vi "Terminal-ModbusEthernet-ReadRegistersWithDateTime.vi"(5 "write operation timeout (ms)":i32=5000 caption="写操作超时（毫秒）", 7 "read operation timeout (ms)":i32=5000 caption="读操作超时（毫秒）", 8 "error in":errorcluster, 9 "number of holding registers":u16 caption="保持寄存器数量", 10 "starting address":u16 caption="起始地址", 11 "unit ID":u8 caption="单元ID") -> (0 "error out":errorcluster, 2 "时间标识":timestamp, 3 "register values":u16[](array[numeric]) caption="寄存器值")   [LabVIEW 2014]
uses:
  <vilib>/Modbus/subvis/Modbus API/Modbus API.lvclass/Modbus API.ctl
  <vilib>/Modbus/subvis/Transmission Data Unit (ADU)/Transmission Data Unit/Transmission Data Unit.lvclass/Transmission Data Unit.ctl
  <vilib>/Modbus/master/Data Access/Unit ID/Set Unit ID Property.vi
  <vilib>/Modbus/subvis/Transmission Data Unit (ADU)/Transmission Data Unit/Data Access/Unit ID/Write Unit ID.vi
  <vilib>/Modbus/subvis/Modbus API/Read Transmission Data Unit.vi
  <vilib>/Modbus/subvis/Modbus API/Write Transmission Data Unit.vi
  Configuration-Global.vi
  <vilib>/Modbus/master/Create Master Instance (TCP).vi
  <vilib>/Modbus/subvis/Transmission Data Unit (ADU)/Transmission Data Unit/Transmission Data Unit.lvclass
  <vilib>/Modbus/master/Modbus Master.lvclass
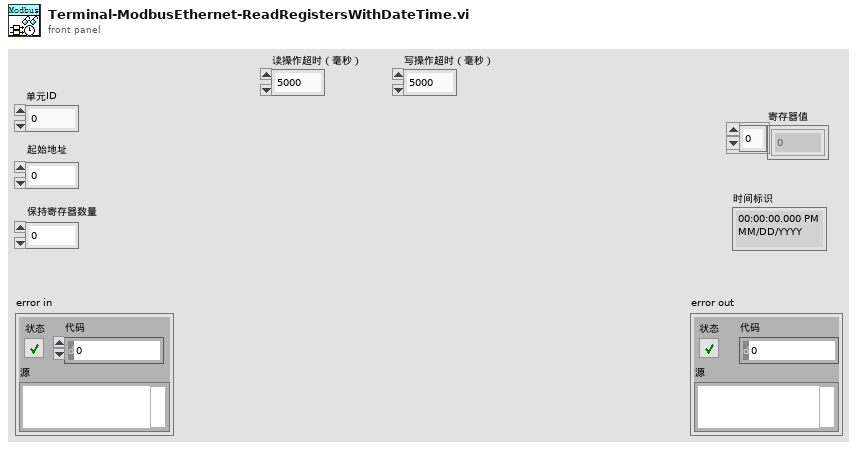
[diagram p1: front panel]
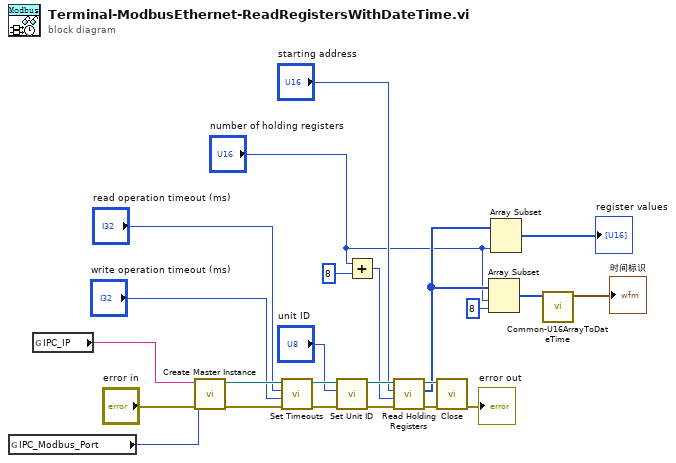
[diagram p0: block diagram]
diagram:
  n1 = global read "Configuration-Global.vi" "IPC_Modbus_Port"() -> (w1:i32)
  n2 = global read "Configuration-Global.vi" "IPC_IP"() -> (w2:string)
  n3 = call-poly <vilib>:"Create Master Instance.vi"("error in (no error)"="error in", "port (502)"=w1, "address"=w2) -> ("error out"=w22:errorcluster, "TCP master instance"=w21:refnum<class "Modbus Master.lvclass">)  [unwired: 7 in]
  n4 = call <vilib>:"Set Timeouts.vi"("error in (no error)"=w22, "write operation timeout (ms)"="write operation timeout (ms)", "read operation timeout (ms)"="read operation timeout (ms)", "Modbus master in"=w21) -> ("error out"=w13:errorcluster, "Modbus master out"=w23:refnum<class "Modbus Master.lvclass">)  [unwired: 6 in]
  n5 = call <vilib>:"Set Unit ID.vi"("error in (no error)"=w13, "unit ID"="unit ID", "Modbus master in"=w23) -> ("error out"=w15:errorcluster, "Modbus master out"=w14:refnum<class "Modbus Master.lvclass">)  [unwired: 7 in]
  n6 = Add(x="number of holding registers", y=u16 8) -> (x+y=w9:u16)
  n7 = call-dynamic "Read Holding Registers.vi"("error in (no error)"=w15, "number of holding registers"=w9, "starting address"="starting address", "Modbus master in"=w14) -> ("error out"=w17:errorcluster, "register values"=w7:u16[], "Modbus master out"=w18:refnum<class "Modbus Master.lvclass">)  [unwired: 5 in]
  n8 = call-dynamic "Close.vi"("error in (no error)"=w17, "Modbus master in"=w18) -> ("error out"=→"error out":errorcluster)  [unwired: 9 in]
  n9 = Array Subset(array=w7, index="number of holding registers", length=8 ("长度")) -> (w4:u16[])
  n10 = Array Subset(array=w7, length="number of holding registers") -> (→"register values":u16[])  [unwired: 1 in]
  n11 = call "Common-U16ArrayToDateTime.vi"("U16Array"=w4) -> ("时间标识"=→"时间标识":timestamp)  [unwired: 10 in]
